vi "CreateFile(IncludeDirectory).vi"(11 "appended path":path) -> (3 "LogFile path输出":path)   [LabVIEW 2018]
doc: "创建文件和目录结构，并返回目录或文件句柄"
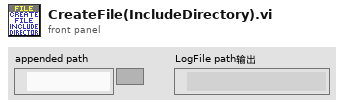
[diagram p1: front panel]
types:
  T1 = enum16{"open", "replace", "create", "open or create", "replace or create", "replace or create with confirmation"}
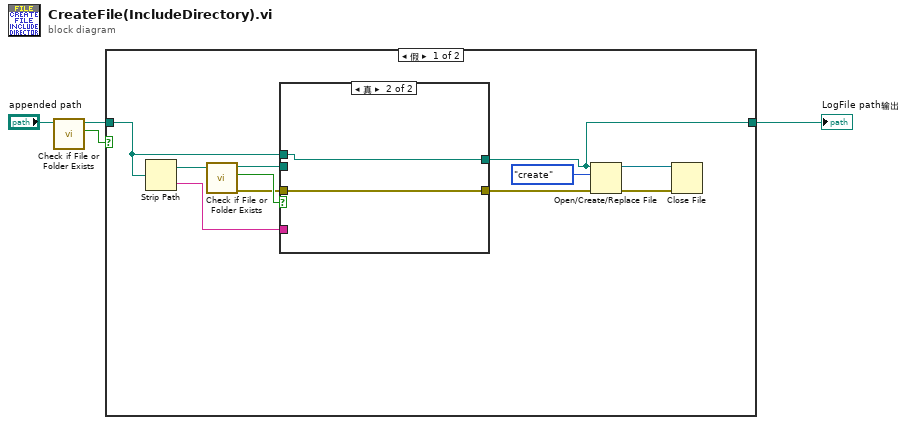
[diagram p0: block diagram]
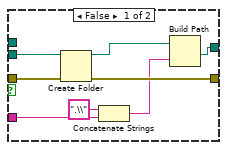
[diagram p2: hidden frame]
diagram:
  n1 = call <vilib>:"Check if File or Folder Exists.vi"("path"="appended path") -> ("file or folder exists?"=w2:bool, "dup path"=w3:path)  [unwired: 8 in, 1 out]
  n2 = case shown="假" w2 {
    tunnel: w3 -> [w11 w26]
    tunnel: [w5 w26] -> w4
    frame False {
      n3 = Strip Path(path=w11) -> (stripped path=w15:path, name=w6:string)
      n4 = call <vilib>:"Check if File or Folder Exists.vi"("path"=w15) -> ("error out"=w12:errorcluster, "file or folder exists?"=w14:bool, "dup path"=w13:path)  [unwired: 8 in]
      n5 = case shown="真" w14 {
        tunnel: w13 -> [w23 _]
        tunnel: w12 -> [w22 w25]
        tunnel: w11 -> [_ w24]
        tunnel: [w21 w25] -> w10
        tunnel: w6 -> [w19 _]
        tunnel: [w16 w24] -> w5
        frame False {
          n6 = Create Folder(path (use dialog)=w23, error in=w22) -> (created path=w20:path, error out=w21:errorcluster)  [unwired: 1 in, 1 out]
          n7 = Concatenate Strings(".\\" ("字符串"), w19) -> (w18:string)
          n8 = Build Path(base path=w20, name or relative path=w18) -> (appended path=w16:path)
        }
        frame True {
        }
      }
      n9 = Open/Create/Replace File(file path (use dialog)=w5, error in=w10, operation (0:open)=T1."create" ("操作(0:open)")) -> (refnum out=w8:refnum<file>, error out=w9:errorcluster)  [unwired: 3 in, 1 out]
      n10 = Close File(refnum=w8, error in=w9) -> ()  [unwired: 2 out]
    }
    frame True {
    }
  }
  "LogFile path输出" <- w4
